vi "Init Device.vi"(8 "error in (no error)":errorcluster, 11 "Camera in":refnum<class "Camera.lvclass">) -> (0 "error out":errorcluster, 3 "Camera out":refnum<class "Camera.lvclass">)   [LabVIEW 2015, in "Camera.lvlib" / "Camera.lvclass"]
uses:
  Camera.lvclass
  Device/Device.lvclass
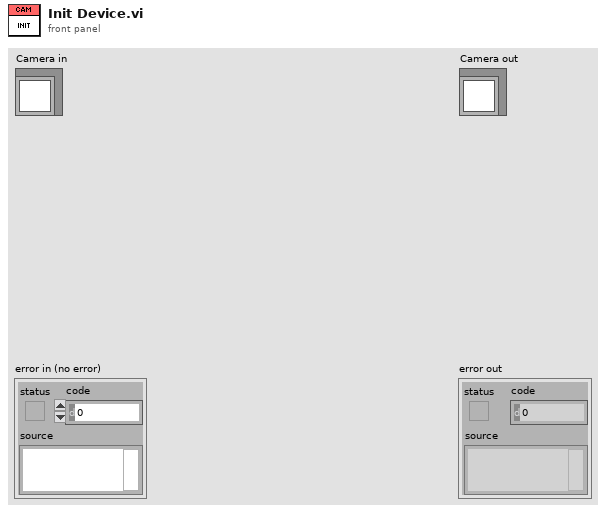
[diagram p1: front panel]
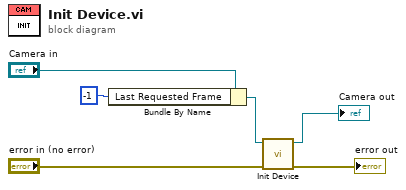
[diagram p0: block diagram]
diagram:
  n1 = Bundle By Name(cluster="Camera in", "Last Requested Frame"=-1) -> (w2:refnum<class "Camera.lvclass">)
  n2 = call-parent "Init Device.vi"("error in (no error)"="error in (no error)", "Device in"=w2) -> ("error out"=→"error out":errorcluster, "Device out"=→"Camera out":refnum<class "Camera.lvclass">)  [unwired: 8 in]
